vi "iViewShutdown.vi"(8 "error in (no error)":errorcluster, 11 "Controller in":refnum<class "Controller.lvclass">) -> (0 "error out":errorcluster, 3 "Controller out":refnum<class "Controller.lvclass">)   [LabVIEW 2020, in "Container.lvlib" / "Controller.lvclass"]
uses:
  Controller.lvclass
  Controller.lvclass/Controller.ctl
  iView/iView.lvclass
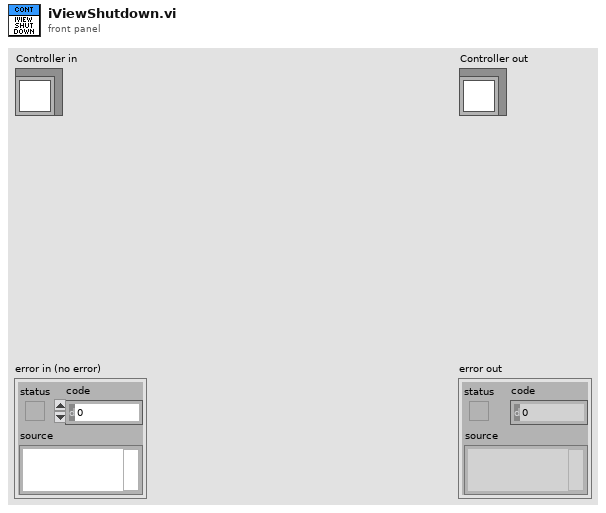
[diagram p1: front panel]
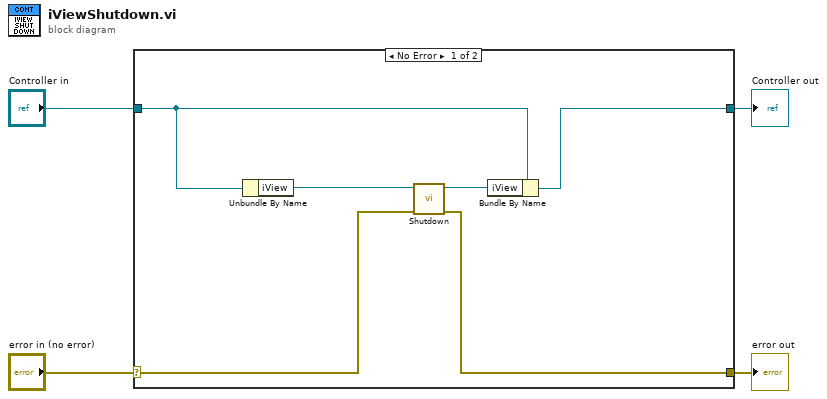
[diagram p0: block diagram]
diagram:
  n1 = case shown="No Error" "error in (no error)" {
    selector: "error in (no error)" -> [w5 w12]
    tunnel: [w8 w12] -> w3
    tunnel: [w9 w11] -> w1
    tunnel: "Controller in" -> [w10 w11]
    frame No Error {
      n2 = Unbundle By Name(w10) -> ("iView"=w6:refnum<class "iView.lvclass">)
      n3 = call-dynamic "Shutdown.vi"("error in (no error)"=w5, "iView in"=w6) -> ("error out"=w8:errorcluster, "iView out"=w7:refnum<class "iView.lvclass">)  [unwired: 8 in]
      n4 = Bundle By Name(cluster=w10, "iView"=w7) -> (w9:refnum<class "Controller.lvclass">)
    }
    frame Error {
    }
  }
  "error out" <- w3
  "Controller out" <- w1
